vi "Create Next or Previous Path.vi"(8 "error in (no error)":errorcluster, 10 "Next?":bool, 11 "current image":path) -> (0 "error out":errorcluster, 2 "file or folder exists?":bool, 3 "next or previous image":path)   [LabVIEW 2014, in "HIJ Vision File Viewer App.lvlib" / "HIJ Vision File Viewer App.lvclass"]
uses:
  HIJ Vision File Viewer App.lvclass
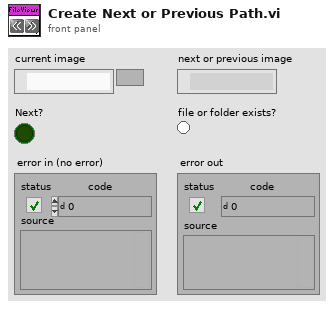
[diagram p1: front panel]
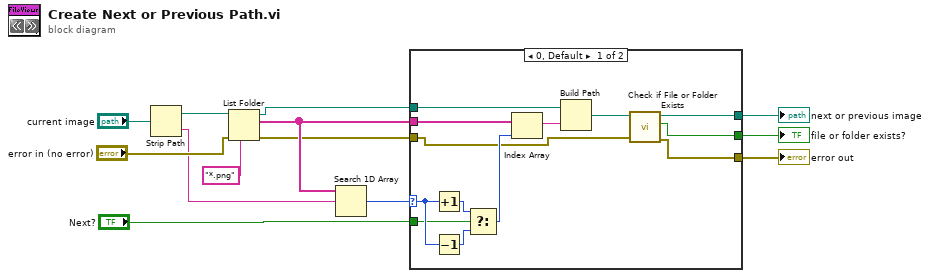
[diagram p0: block diagram]
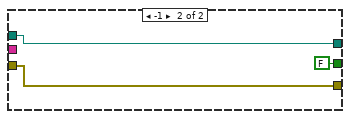
[diagram p2: hidden frame]
diagram:
  n1 = Strip Path(path="current image") -> (stripped path=w12:path, name=w10:string)
  n2 = List Folder(path=w12, pattern="*.png", error in="error in (no error)") -> (path out=w6:path, filenames=w7:string[], error out=w3:errorcluster)  [unwired: 1 in, 1 out]
  n3 = Search 1D Array(1D array=w7, element=w10) -> (index of element=w9:i32)  [unwired: 1 in]
  n4 = case shown="0, Default" w9 {
    selector: w9 -> [w25 _]
    tunnel: "Next?" -> [w24 _]
    tunnel: w7 -> [w26 _]
    tunnel: w6 -> [w19 w29]
    tunnel: [w15 w29] -> w5
    tunnel: [w17 w28] -> w4
    tunnel: w3 -> [w18 w28]
    tunnel: [w14 FALSE ("file or folder exists?")] -> w2
    frame 0, Default {
      n5 = Increment(x=w25) -> (x+1=w23:i32)
      n6 = Decrement(x=w25) -> (x-1=w22:i32)
      n7 = Select(t=w23, s=w24, f=w22) -> (s? t:f=w21:i32)
      n8 = Index Array(array=w26, index=w21) -> (element=w20:string)
      n9 = Build Path(base path=w19, name or relative path=w20) -> (appended path=w16:path)
      n10 = call <vilib>:"Check if File or Folder Exists.vi"("error in (no error)"=w18, "path"=w16) -> ("error out"=w17:errorcluster, "file or folder exists?"=w14:bool, "dup path"=w15:path)  [unwired: 7 in]
    }
    frame -1 {
    }
  }
  "next or previous image" <- w5
  "error out" <- w4
  "file or folder exists?" <- w2
